vi "Save_sequences.vi"(0 "Sequences":T1(array[cluster])) -> ()   [LabVIEW 2016]
uses:
  <vilib>/Utility/xml.llb/Write to XML File(string).vi
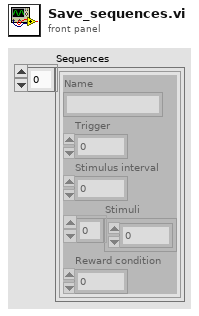
[diagram p1: front panel]
types:
  T1 = cluster{"Name":string, "Trigger":u16, "Stimulus interval":dbl, "Stimuli":i32[], "Reward condition":u16}[]
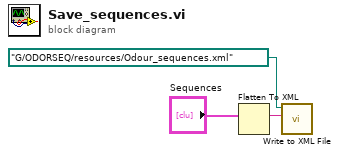
[diagram p0: block diagram]
diagram:
  n1 = Flatten To XML(anything="Sequences") -> (xml string=w2:string)
  n2 = call-poly <vilib>:"Write to XML File.vi"("XML Input"=w2, "XML File Path"=path "G:/ODORSEQ/resources/Odour_sequences.xml") -> ()  [unwired: 7 in, 3 out]
